vi "RT Main.vi"() -> ()   [LabVIEW 2018]
uses:
  <vilib>/DAQmx/read.llb/DAQmx Read.vi
  <vilib>/DAQmx/read.llb/DAQmx Read (Analog 1D Wfm NChan NSamp).vi
  <vilib>/DAQmx/miscellaneous.llb/DAQmx Fill In Error Info.vi
  <vilib>/NI_Real-Time Target Support.lvlib
panel:
  out "CPU Load":dbl(graph)
  out "Data":dbl[](array[numeric])
  in  "stop":bool
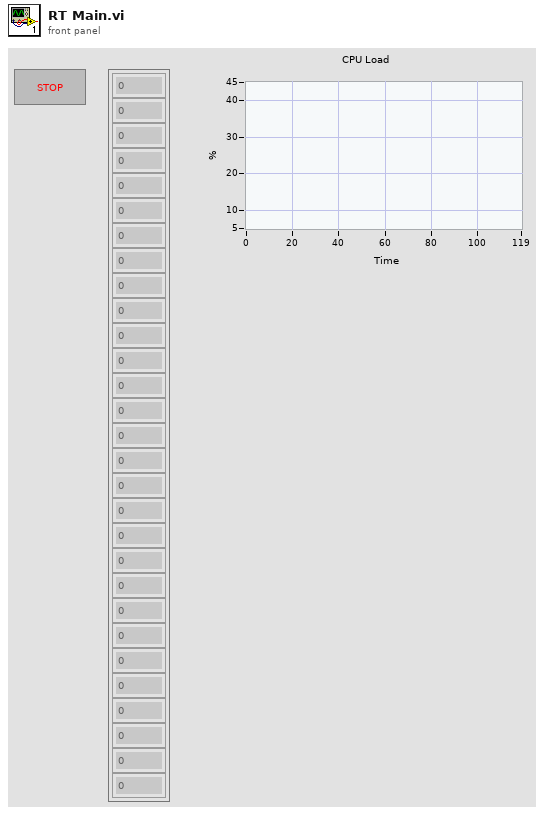
[diagram p1: front panel]
types:
  T1 = typedef "NI_Real-Time Target Support.lvlib/RT CPU Load.ctl" = cluster{"Total (%)":dbl, "Time Critical (%)":dbl, "Timed Structures (%)":dbl, "High (%)":dbl, "Above Normal (%)":dbl, "Normal (%)":dbl, "Background (%)":dbl, "Idle (%)":dbl, "ISR (%)":dbl}
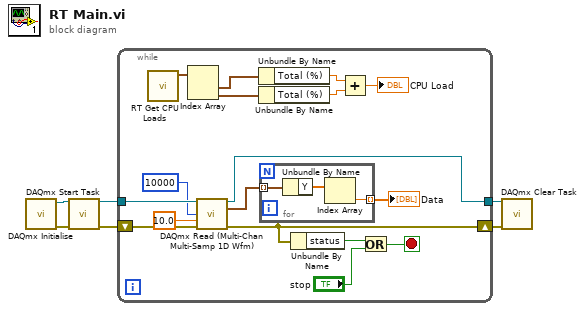
[diagram p0: block diagram]
diagram:
  n1 = call "DAQmx Initialise.vi"() -> ("error out"=w1:errorcluster, "task out"=w2:refnum<k21>)  [unwired: 10 in]
  n2 = call <vilib>:"DAQmx Start Task.vi"("task/channels in"=w2, "error in"=w1) -> ("task out"=w6:refnum<k21>, "error out"=w5:errorcluster)  [unwired: 12 in]
  n3 = while {
    tunnel: w6 -> [w23]
    tunnel: [w21] -> w3
    shift-right: [w19] -> w4
    shift-left: w5 -> [w22]
    stop <- w18 stop-if-true
    n4 = call <vilib>:"RT Get CPU Loads.vi"() -> ("CPU loads"=w13:T1[])  [unwired: 10 in, 1 out]
    n5 = Index Array(array=w13) -> (element #1=w12:T1, element #2=w11:T1)  [unwired: 2 in]
    n6 = call-poly "DAQmx Read (Multi-Chan Multi-Samp 1D Wfm).vi"("task/channels in"=w23, "number of samples per channel"=10000 ("number of samples"), "timeout"=10.0 ("timeout (s)"), "error in"=w22) -> ("task out"=w21:refnum<k21>, "data"=w15:waveform(dbl)[], "error out"=w19:errorcluster)  [unwired: 9 in]
    n7 = Unbundle By Name(w12) -> ("Total (%)"=w10:dbl)
    n8 = Unbundle By Name(w11) -> ("Total (%)"=w9:dbl)
    n9 = for {
      tunnel: w15 -> [w26] mode=indexing
      tunnel: [w24] -> w14 mode=indexing
      n10 = Unbundle By Name(w26) -> ("Y"=w25:dbl[])
      n11 = Index Array(array=w25) -> (element=w24:dbl)  [unwired: 1 in]
    }
    "Data" <- w14
    n12 = Unbundle By Name(w19) -> ("status"=w20:bool)
    n13 = Add(x=w10, y=w9) -> (x+y=→"CPU Load":dbl)
    n14 = Or(x=w20, y="stop") -> (x .or. y?=w18:bool)
  }
  n15 = call <vilib>:"DAQmx Clear Task.vi"("task in"=w3, "error in"=w4) -> ()  [unwired: 13 in, 1 out]
